vi "test5.vi"() -> ()   [LabVIEW 2018]
uses:
  <vilib>/imath/engines/lvmath2/RunTimeEngine/BuiltInFunctions/randnormal/NIMS_randnormal(1,I32).vi
  <vilib>/imath/engines/lvmath2/RunTimeEngine/ErrorHandling/NIMS_Error From Error Code.vi
  <vilib>/imath/engines/lvmath2/RunTimeEngine/RangeToken/NIMS_Range.vi
  <instcachedir>/0/NIMS_Range_846134F467D14A349F7C6CCEF459CDB2.lvgen/NIMS_Range_846134F467D14A349F7C6CCEF459CDB2_000.vi
  <vilib>/imath/engines/lvmath2/RunTimeEngine/IndexReplace/NIMS V(V)=M.vi
  <instcachedir>/0/NIMS V(V)=M_557AD341475A438FADE1C41F5251DF67.lvgen/NIMS V(V)=M_557AD341475A438FADE1C41F5251DF67_001.vi
  <vilib>/imath/engines/lvmath2/RunTimeSupport/NIMS_Error if Not Equal.vi
  <instcachedir>/0/NIMS_Error if Not Equal_C77461FADD9B4AE6B0EA3ED6E3A6D94D.lvgen/NIMS_Error if Not Equal_C77461FADD9B4AE6B0EA3ED6E3A6D94D_001.vi
  <vilib>/imath/engines/lvmath2/RunTimeEngine/ErrorHandling/NIMS_Create Error From Enums.vi
  <vilib>/imath/engines/lvmath2/RunTimeEngine/BuiltInFunctions/crosscorr/NIMS_crosscorr(GV,GV,Str).vi
  <instcachedir>/0/NIMS_crosscorr(GV,GV,Str)_A4EB815E9E924C97804DA22507CDE303.lvgen/NIMS_crosscorr(GV,GV,Str)_A4EB815E9E924C97804DA22507CDE303_001.vi
  <vilib>/imath/engines/lvmath2/RunTimeEngine/BuiltInFunctions/max/1 input/NIMS_max(CV).vi
  <instcachedir>/0/NIMS_max(CV)_55667A76FB394995B16030C4321F839C.lvgen/NIMS_max(CV)_55667A76FB394995B16030C4321F839C_000.vi
  <vilib>/imath/engines/lvmath2/RunTimeEngine/BuiltInFunctions/abs/NIMS_abs(signed).vi
  <instcachedir>/0/NIMS_abs(signed)_C4FCB8E6058B49B797C7C8D53CA5F6EC.lvgen/NIMS_abs(signed)_C4FCB8E6058B49B797C7C8D53CA5F6EC_000.vi
  <vilib>/imath/engines/lvmath2/RunTimeEngine/IndexReplace/NIMS V(R2)=M.vi
  <instcachedir>/0/NIMS V(R2)=M_F16E001901484C228445F92C266A8F4F.lvgen/NIMS V(R2)=M_F16E001901484C228445F92C266A8F4F_000.vi
  <vilib>/imathl/engines/lvmath/Functions/Error Handling/Create Error.vi
  <instcachedir>/0/NIMS V(V)=M_557AD341475A438FADE1C41F5251DF67.lvgen/NIMS V(V)=M_557AD341475A438FADE1C41F5251DF67_002.vi
  <instcachedir>/0/NIMS V(R2)=M_F16E001901484C228445F92C266A8F4F.lvgen/NIMS V(R2)=M_F16E001901484C228445F92C266A8F4F_001.vi
  <vilib>/imath/engines/lvmath2/RunTimeEngine/NodeEndStatement/NIMS_NodeEndStatement_Output.vi
  <instcachedir>/0/NIMS_NodeEndStatement_Output_53EC0D466D134D7ABD903AC30B43404B.lvgen/NIMS_NodeEndStatement_Output_53EC0D466D134D7ABD903AC30B43404B_005.vi
  <instcachedir>/0/NIMS_NodeEndStatement_Output_53EC0D466D134D7ABD903AC30B43404B.lvgen/NIMS_NodeEndStatement_Output_53EC0D466D134D7ABD903AC30B43404B_000.vi
  <instcachedir>/0/NIMS_NodeEndStatement_Output_53EC0D466D134D7ABD903AC30B43404B.lvgen/NIMS_NodeEndStatement_Output_53EC0D466D134D7ABD903AC30B43404B_001.vi
  <vilib>/imath/engines/lvmath2/RunTimeEngine/ErrorHandling/NIMS_Finalize Error.vi
panel:
  out "XY Graph":cluster{"x":dbl[], "xlags":dbl[]}(graph)
  out "Tlag":dbl
  in  "lag":dbl=40.0
  in  "num":dbl=10000.0
  in  "a":dbl=4.0
  in  "mn":dbl=1.0
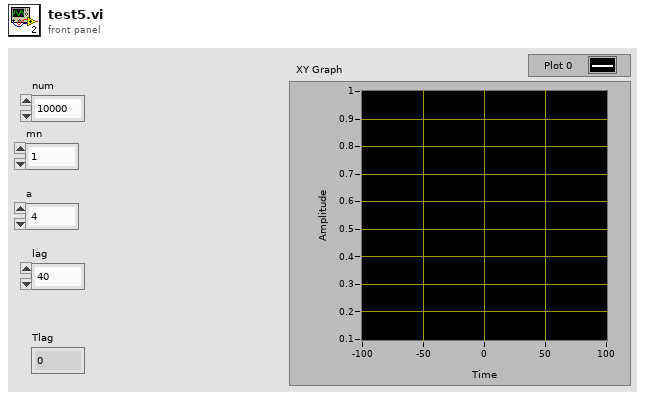
[diagram p1: front panel]
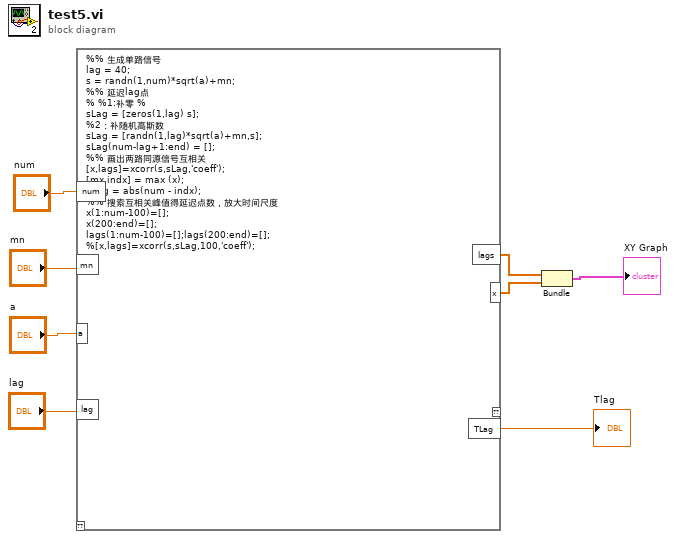
[diagram p0: block diagram]
diagram:
  n1 = mathscript code="%% 生成单路信号\nlag = 40;\ns = randn(1,num)*sqrt(a)+mn;\n%% 延迟lag点\n% %1:补零 % \nsLag = [zeros(1,lag) s]; \n%2：补随机高斯数\nsLag = [randn(1,lag)*sqrt(a)+mn,s];\nsLag(num-lag+1:end) = [];\n%% 画出两路同源信号互相关\n[x,lags]=xcorr(s,sLag,'coeff');\n[mx,indx] = max (x);\nTLag = abs(num - indx);\n%% 搜索互相关峰值得延迟点数，放大时间尺度\nx(1:num-100)=[];\nx(200:end)=[];\nlags(1:num-100)=[];lags(200:end)=[];\n%[x,lags]=xcorr(s,sLag,100,'coeff');"("num"="num", "mn"="mn", "a"="a", "lag"="lag") -> ("TLag"=→"Tlag":dbl, "x"=w1:cdb[], "lags"=w2:dbl[])  [unwired: 1 in, 1 out]
  n2 = Bundle("lags"=w2, "x"=w1) -> (→"XY Graph":cluster{"lags":dbl[], "x":cdb[]})  [unwired: 1 in]
